vi "ErrorMSG_Panel timeout.vi"(6 "Timeout":u32=10000, 8 "error in (no error)":errorcluster, 10 "reference":refnum<vi>, 11 "String":string) -> (0 "error out":errorcluster, 3 "Timeout":bool)   [LabVIEW 2019]
uses:
  <vilib>/Utility/miscctls.llb/LVPointTypeDef.ctl
panel:
  out "Slide":u8(slide) max=10 scale=0.0..100.0
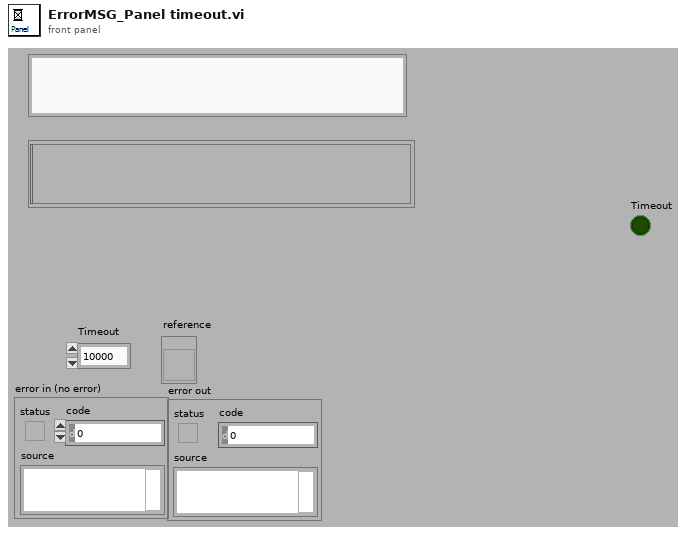
[diagram p1: front panel]
types:
  T1 = typedef "LVPointTypeDef.ctl" = cluster{"Horizontal":i16, "Vertical":i16}
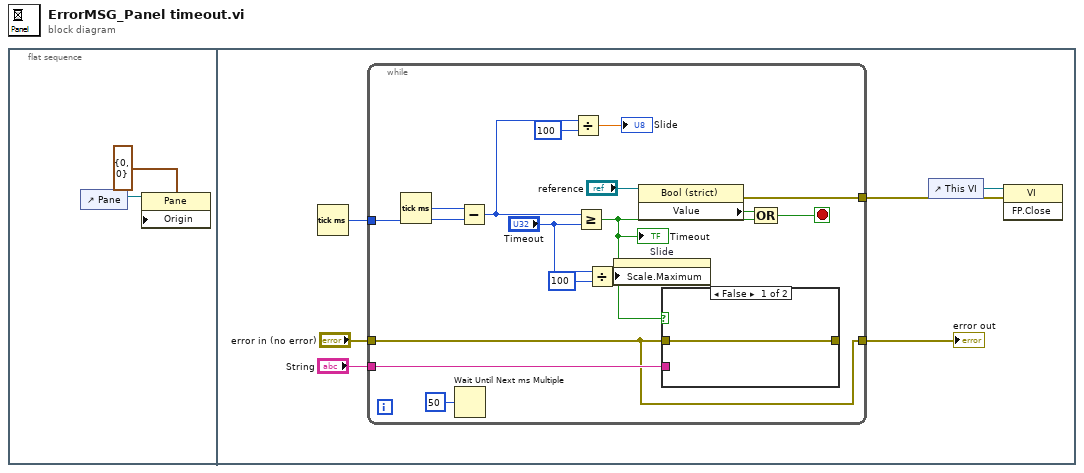
[diagram p0: block diagram]
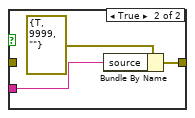
[diagram p2: hidden frame]
diagram:
  n1 = flat-sequence {
    frame #0 {
      n2 = control-ref of="Pane"() -> (w2:refnum<vi>)
      n3 = property class="Pane"(reference=w2, "Origin"=T1 {"Horizontal"=0, "Vertical"=0}) -> ()  [unwired: 1 in, 2 out]
    }
    frame #1 {
      n4 = Tick Count (ms)() -> (millisecond timer value=w8:u32)
      n5 = while {
        tunnel: w8 -> [w22]
        tunnel: "error in (no error)" -> [w9]
        tunnel: [w9] -> w6
        tunnel: "String" -> [w11]
        tunnel: [w10] -> w3
        stop <- w15 stop-if-true
        n6 = Tick Count (ms)() -> (millisecond timer value=w23:u32)
        n7 = Wait Until Next ms Multiple(millisecond multiple=u32 50) -> ()  [unwired: 1 out]
        n8 = Subtract(x=w23, y=w22) -> (x-y=w17:u32)
        n9 = Divide(x=w17, y=u32 100) -> (x/y=→"Slide":dbl)
        n10 = Greater Or Equal?(x=w17, y="Timeout") -> (x >= y?=w12:bool)
        "Timeout" <- w12
        n11 = Divide(x="Timeout", y=u32 100) -> (x/y=w20:dbl)
        n12 = property on="Slide" class="Slide (strict)"("Scale.Maximum"=w20) -> ()  [unwired: 2 in, 2 out]
        n13 = property class="Bool (strict)"(reference="reference") -> (error out=w10:errorcluster, "Value"=w14:bool)  [unwired: 1 in, 1 out]
        n14 = case shown="False" w12 {
          tunnel: w9 -> [w25 _]
          tunnel: [w25 w27] -> _
          tunnel: w11 -> [_ w26]
          frame False {
          }
          frame True {
            n15 = Bundle By Name(cluster=errorcluster {"status"=TRUE, "code"=9999, "source"=""} ("error in (no error)"), "source"=w26) -> (w27:errorcluster)
          }
        }
        n16 = Compound Arithmetic op=OR(w14, w12) -> (w15:bool)
      }
      "error out" <- w6
      n17 = control-ref of="This VI"() -> (w4:refnum<vi>)
      n18 = invoke class="VI" method="FP.Close"(reference=w4, error in=w3) -> ()  [unwired: 1 in, 3 out]
    }
  }
